vi "Dashboard Main.vi"() -> ()   [LabVIEW 2013]
uses:
  Downloads/Control 1.ctl
  <vilib>/event_ctls.llb/eventvkey.ctl
  <vilib>/Utility/file.llb/Read From Spreadsheet File (DBL).vi
panel:
  in  "Tab Control":T1(tab)
  out "Loaded":T2
  out "Armed":T2
  out "Gathering":T2
  out "Gyro":T2
  out "Flip Axes":T2
  out "Winch Power":T2
  out "Offset":dbl format="Offset: %#_g"
  out "Shot count":dbl format="%#_g shots"
  out "Offset Recieved":dbl
  in  "Jew Bar":bool=TRUE
  in  "Arm":bool=TRUE
  in  "Winch":bool=TRUE
  in  "Trigger":bool=TRUE
  in  "Intake":bool=TRUE
  in  "Rollers":bool=TRUE
  in  "Right Drive":bool=TRUE
  in  "Left Drive":bool=TRUE
  in  "Close KnightVision":bool
  in  "Open KnightVision":bool
  out "Mode":string
  out "Vision":string
  out "data out":string
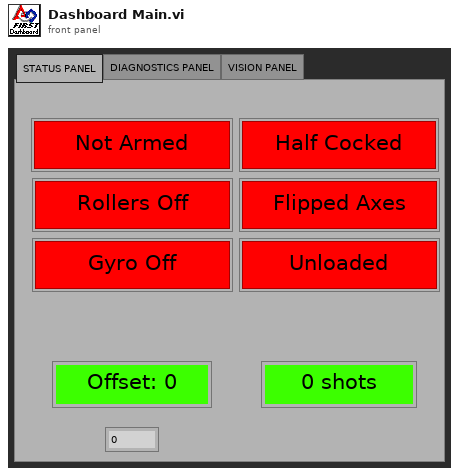
[diagram p1: front panel]
types:
  T1 = enum32{"STATUS PANEL", "DIAGNOSTICS PANEL", "VISION PANEL"}
  T2 = typedef "Control 1.ctl" = bool
  T3 = typedef "eventvkey.ctl" = enum16{"ASCII", "Enter", "Return", "Shift", "Ctrl", "Alt", "Cmd", "Opt", "Caps", "NumLock", "Clear", "Break", "Up", "Down", "Left", "Right", "Insert", "Delete", "Home", "End", "PageUp", "PageDown", "Escape", "Help", "Pause", "ScrollLock", "F1", "F2", "F3", "F4", "F5", "F6", "F7", "F8", "F9", "F10", "F11", "F12", "F13", "F14", "F15", "F16", "F17", "F18", "F19", "F20", "F21", "F22", "F23", "F24", "Play", "VolumeUp", "VolumeDown", "Mute", "Two Byte Char"}
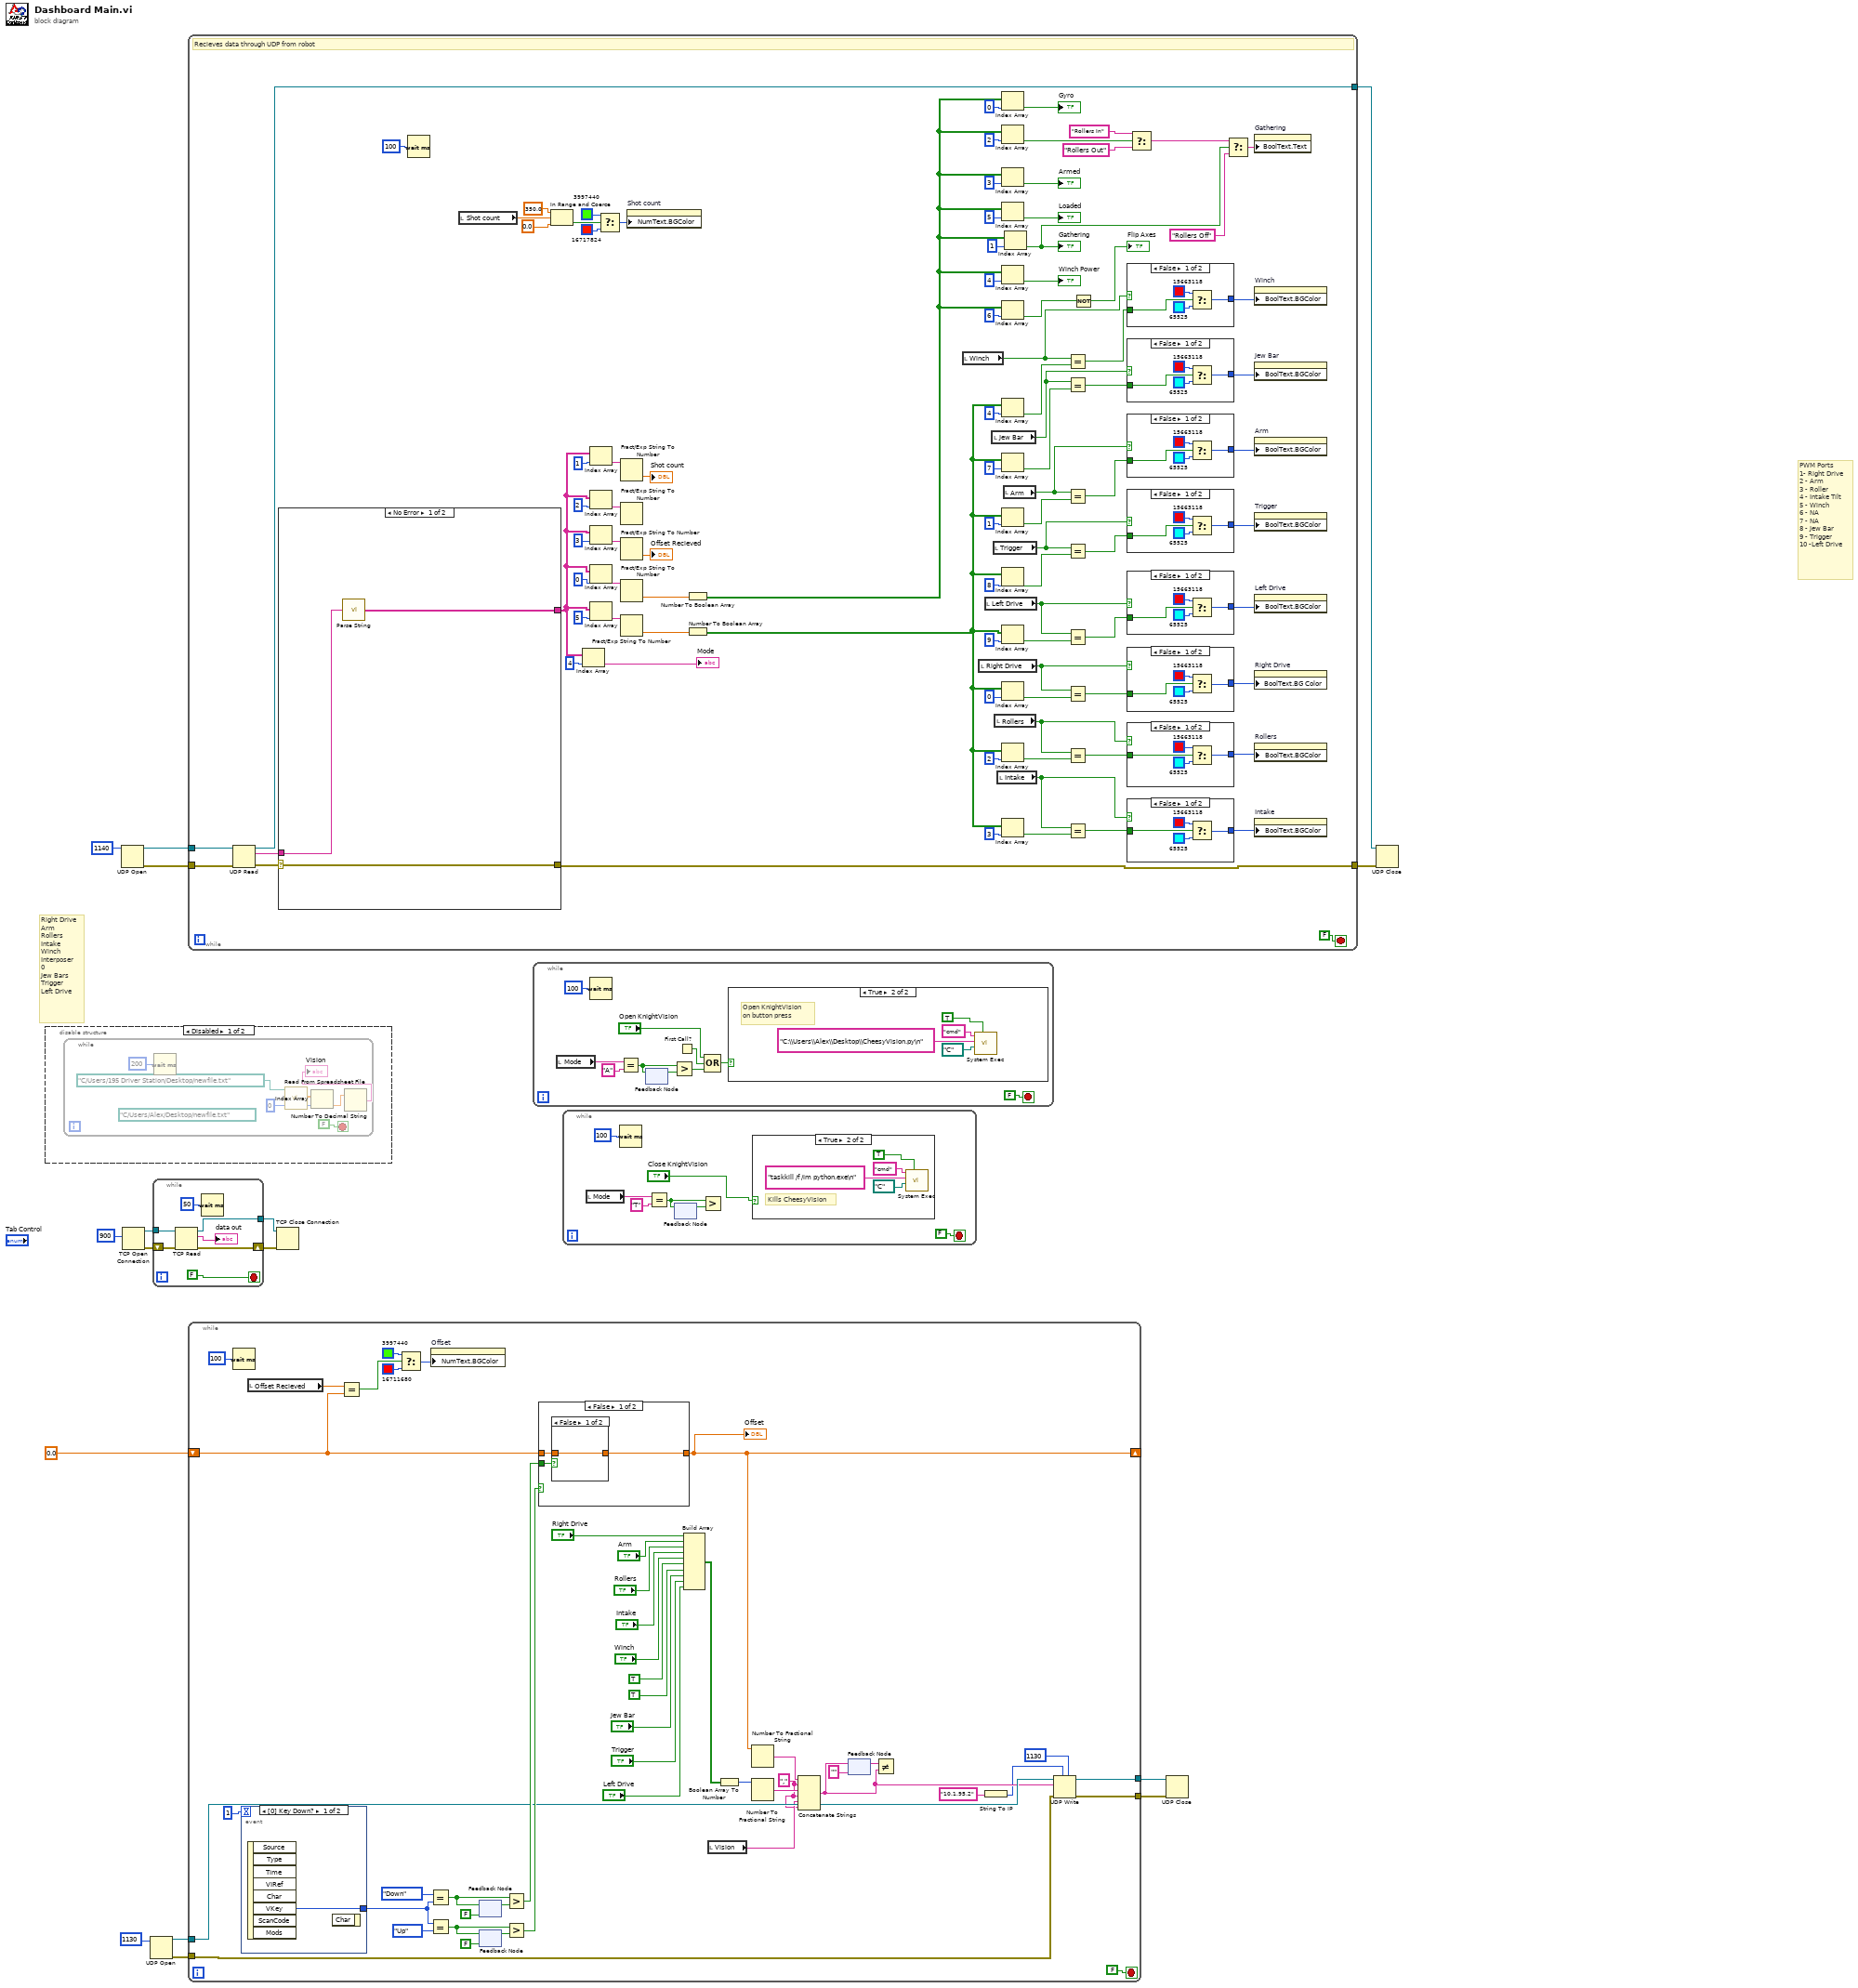
[diagram p0: block diagram]
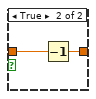
[diagram p5: hidden frame]
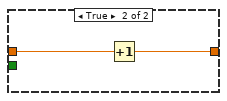
[diagram p6: hidden frame]
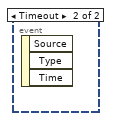
[diagram p7: hidden frame]
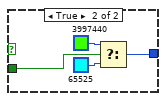
[diagram p8: hidden frame]
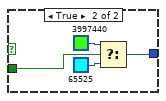
[diagram p9: hidden frame]
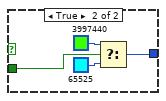
[diagram p10: hidden frame]
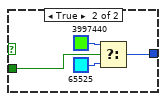
[diagram p11: hidden frame]
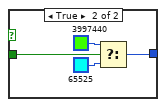
[diagram p12: hidden frame]
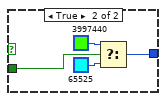
[diagram p13: hidden frame]
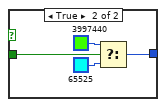
[diagram p14: hidden frame]
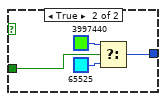
[diagram p15: hidden frame]
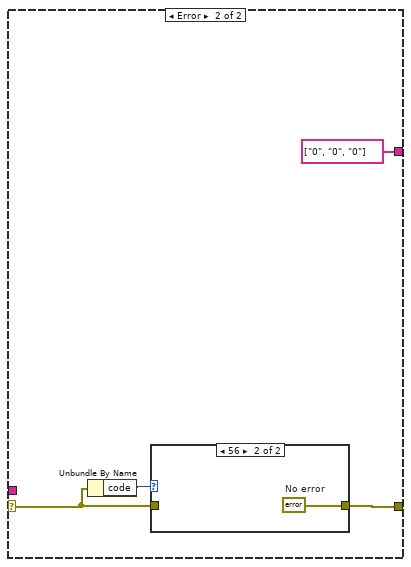
[diagram p16: hidden frame]
diagram:
  # "PWM Ports\n1- Right Drive\n2 - Arm\n3 - Roller\n4 - Intake Tilt \n5 - Winch\n6 - NA \n7 - NA\n8 - Jew Bar\n9 - Trigger\n10 -Left Drive"
  # "Right Drive\nArm\nRollers\nIntake\nWinch\nInterposer\n0\nJew Bars\nTrigger\nLeft Drive"
  n1 = disable-structure shown="Disabled" {
    frame Disabled {
      n2 = while {
        stop <- FALSE stop-if-true
        (unwired) path "C:/Users/Alex/Desktop/newfile.txt" ("file (use dialog)")
        n3 = Wait (ms)(milliseconds to wait=u32 200) -> ()  [unwired: 1 out]
        n4 = call-poly <vilib>:"Read From Spreadsheet File.vi"("file path (dialog if empty)"=path "C:/Users/195 Driver Station/Desktop/newfile.txt" ("file (use dialog)")) -> ("first row"=w21:dbl[])  [unwired: 6 in, 4 out]
        n5 = Index Array(array=w21, index=0) -> (element=w19:dbl)
        n6 = Number To Decimal String(number=w19) -> (decimal integer string=→"Vision":string)  [unwired: 1 in]
      }
    }
    frame Enabled {
    }
  }
  n7 = UDP Open(11:u16 1140) -> (port=w13:refnum<k16>, 0:w14:errorcluster)  [unwired: 4 in, 1 out]
  n8 = TCP Open Connection(remote port or service name=u16 900) -> (connection ID=w3:refnum<k5>, error out=w2:errorcluster)  [unwired: 4 in]
  n9 = UDP Open(11:u16 1130 ("port")) -> (port=w9:refnum<k16>, 0:w8:errorcluster)  [unwired: 4 in, 1 out]
  n10 = while {
    tunnel: [w29] -> w5
    tunnel: w3 -> [w27]
    shift-right: [w28] -> w4
    shift-left: w2 -> [w26]
    stop <- FALSE stop-if-true
    n11 = TCP Read(connection ID=w27, error in (no error)=w26) -> (connection ID out=w29:refnum<k5>, data out=→"data out":string, error out=w28:errorcluster)  [unwired: 3 in]
    n12 = Wait (ms)(milliseconds to wait=u32 50) -> ()  [unwired: 1 out]
  }
  n13 = while {
    tunnel: [w124] -> w16
    tunnel: [w123] -> w15
    tunnel: w14 -> [w122]
    tunnel: w13 -> [w121]
    stop <- FALSE stop-if-true
    # "Recieves data through UDP from robot"
    n14 = UDP Read(connection ID=w121, 8:w122) -> (data out=w120:string, error out=w119:errorcluster, 3:w124:refnum<k16>)  [unwired: 1 in, 3 out]
    n15 = case shown="No Error" w119 {
      selector: w119 -> [w191 w194]
      tunnel: w120 -> [w190 _]
      tunnel: [w191 w193] -> w123
      tunnel: [w189 string[] ["0", "0", "0"] ("Array Out")] -> w33
      frame No Error {
        n16 = call "Parse String.vi"("String In"=w190) -> ("Array Out"=w189:string[])
      }
      frame Error {
        n17 = Unbundle By Name(w194) -> ("code"=w195:i32)
        n18 = case shown="56" w195 {
          tunnel: w194 -> [w196 _]
          tunnel: [w196 w197] -> w193
          frame Default {
          }
          frame 56 {
            w197 = errorcluster {"status"=FALSE, "code"=0, "source"=""}  # No error
          }
        }
      }
    }
    n19 = Wait (ms)(milliseconds to wait=u32 100) -> ()  [unwired: 1 out]
    n20 = local read "Shot count"() -> (w94:dbl)
    n21 = In Range and Coerce(upper limit=350.0, x=w94, lower limit=0.0) -> (In Range?=w91:bool)  [unwired: 1 out]
    n22 = Index Array(array=w33, index=4) -> (element=→"Mode":string)
    n23 = Index Array(array=w33, index=1) -> (element=w98:string)
    n24 = Index Array(array=w33, index=2) -> (element=w99:string)
    n25 = Index Array(array=w33, index=3) -> (element=w80:string)
    n26 = Index Array(array=w33, index=0) -> (element=w116:string)
    n27 = Index Array(array=w33, index=5) -> (element=w75:string)
    n28 = Select(t=u32 3997440, s=w91, f=u32 16717824) -> (s? t:f=w78:u32)
    n29 = Fract/Exp String To Number(string=w98) -> (number=→"Shot count":dbl)  [unwired: 3 in, 1 out]
    n30 = Fract/Exp String To Number(string=w99) -> ()  [unwired: 3 in, 2 out]
    n31 = Fract/Exp String To Number(string=w80) -> (number=→"Offset Recieved":dbl)  [unwired: 3 in, 1 out]
    n32 = Fract/Exp String To Number(string=w116) -> (number=w115:dbl)  [unwired: 3 in, 1 out]
    n33 = Fract/Exp String To Number(string=w75) -> (number=w76:dbl)  [unwired: 3 in, 1 out]
    n34 = property on="Shot count" class="DigNum (strict)"("NumText.BGColor"=w78) -> ()  [unwired: 2 in, 2 out]
    n35 = Number To Boolean Array(number=w115) -> (Boolean array=w102:bool[])
    n36 = Number To Boolean Array(number=w76) -> (Boolean array=w37:bool[])
    n37 = local read "Winch"() -> (w32:bool)
    n38 = local read "Right Drive"() -> (w65:bool)
    n39 = local read "Left Drive"() -> (w42:bool)
    n40 = local read "Jew Bar"() -> (w48:bool)
    n41 = local read "Trigger"() -> (w45:bool)
    n42 = local read "Rollers"() -> (w64:bool)
    n43 = local read "Intake"() -> (w60:bool)
    n44 = Index Array(array=w102, index=0) -> (element=→"Gyro":bool)
    n45 = Index Array(array=w102, index=2) -> (element=w83:bool)
    n46 = Index Array(array=w102, index=3) -> (element=→"Armed":bool)
    n47 = Index Array(array=w102, index=5) -> (element=→"Loaded":bool)
    n48 = Index Array(array=w102, index=4) -> (element=→"Winch Power":bool)
    n49 = Index Array(array=w102, index=6) -> (element=w101:bool)
    n50 = Index Array(array=w37, index=4) -> (element=w51:bool)
    n51 = Index Array(array=w37, index=7) -> (element=w47:bool)
    n52 = Index Array(array=w37, index=1) -> (element=w58:bool)
    n53 = Index Array(array=w37, index=8) -> (element=w36:bool)
    n54 = Index Array(array=w37, index=9) -> (element=w35:bool)
    n55 = Index Array(array=w37, index=0) -> (element=w68:bool)
    n56 = Index Array(array=w37, index=2) -> (element=w56:bool)
    n57 = Index Array(array=w37, index=3) -> (element=w52:bool)
    n58 = local read "Arm"() -> (w61:bool)
    n59 = Index Array(array=w102, index=1) -> (element=w82:bool)
    "Gathering" <- w82
    n60 = Equal?(x=w32, y=w51) -> (x = y?=w53:bool)
    n61 = Equal?(x=w48, y=w47) -> (x = y?=w49:bool)
    n62 = Equal?(x=w61, y=w58) -> (x = y?=w62:bool)
    n63 = Equal?(x=w45, y=w36) -> (x = y?=w44:bool)
    n64 = Equal?(x=w42, y=w35) -> (x = y?=w43:bool)
    n65 = Equal?(x=w65, y=w68) -> (x = y?=w67:bool)
    n66 = Equal?(x=w64, y=w56) -> (x = y?=w63:bool)
    n67 = Equal?(x=w60, y=w52) -> (x = y?=w59:bool)
    n68 = Not(x=w101) -> (.not. x?=→"Flip Axes":bool)
    n69 = case shown="False" w32 {
      tunnel: w53 -> [w151 w156]
      tunnel: [w152 w153] -> w50
      frame False {
        n70 = Select(t=u32 15663118, s=w151, f=u32 65525) -> (s? t:f=w152:u32)
      }
      frame True {
        n71 = Select(t=u32 3997440, s=w156, f=u32 65525) -> (s? t:f=w153:u32)
      }
    }
    n72 = case shown="False" w48 {
      tunnel: w49 -> [w143 w148]
      tunnel: [w144 w145] -> w46
      frame False {
        n73 = Select(t=u32 15663118, s=w143, f=u32 65525) -> (s? t:f=w144:u32)
      }
      frame True {
        n74 = Select(t=u32 3997440, s=w148, f=u32 65525) -> (s? t:f=w145:u32)
      }
    }
    n75 = case shown="False" w61 {
      tunnel: w62 -> [w167 w172]
      tunnel: [w168 w169] -> w57
      frame False {
        n76 = Select(t=u32 15663118, s=w167, f=u32 65525) -> (s? t:f=w168:u32)
      }
      frame True {
        n77 = Select(t=u32 3997440, s=w172, f=u32 65525) -> (s? t:f=w169:u32)
      }
    }
    n78 = case shown="False" w45 {
      tunnel: w44 -> [w135 w140]
      tunnel: [w136 w137] -> w41
      frame False {
        n79 = Select(t=u32 15663118, s=w135, f=u32 65525) -> (s? t:f=w136:u32)
      }
      frame True {
        n80 = Select(t=u32 3997440, s=w140, f=u32 65525) -> (s? t:f=w137:u32)
      }
    }
    n81 = case shown="False" w42 {
      tunnel: w43 -> [w127 w132]
      tunnel: [w128 w129] -> w40
      frame False {
        n82 = Select(t=u32 15663118, s=w127, f=u32 65525) -> (s? t:f=w128:u32)
      }
      frame True {
        n83 = Select(t=u32 3997440, s=w132, f=u32 65525) -> (s? t:f=w129:u32)
      }
    }
    n84 = case shown="False" w65 {
      tunnel: w67 -> [w183 w188]
      tunnel: [w184 w185] -> w66
      frame False {
        n85 = Select(t=u32 15663118, s=w183, f=u32 65525) -> (s? t:f=w184:u32)
      }
      frame True {
        n86 = Select(t=u32 3997440, s=w188, f=u32 65525) -> (s? t:f=w185:u32)
      }
    }
    n87 = case shown="False" w64 {
      tunnel: w63 -> [w175 w180]
      tunnel: [w176 w177] -> w55
      frame False {
        n88 = Select(t=u32 15663118, s=w175, f=u32 65525) -> (s? t:f=w176:u32)
      }
      frame True {
        n89 = Select(t=u32 3997440, s=w180, f=u32 65525) -> (s? t:f=w177:u32)
      }
    }
    n90 = case shown="False" w60 {
      tunnel: w59 -> [w159 w164]
      tunnel: [w160 w161] -> w54
      frame False {
        n91 = Select(t=u32 15663118, s=w159, f=u32 65525) -> (s? t:f=w160:u32)
      }
      frame True {
        n92 = Select(t=u32 3997440, s=w164, f=u32 65525) -> (s? t:f=w161:u32)
      }
    }
    n93 = Select(t="Rollers In" ("Boolean Text.Text"), s=w83, f="Rollers Out" ("Boolean Text.Text")) -> (s? t:f=w84:string)
    n94 = Select(t=w84, s=w82, f="Rollers Off") -> (s? t:f=w88:string)
    n95 = property on="Gathering" class="Bool (strict)"("BoolText.Text"=w88) -> ()  [unwired: 2 in, 2 out]
    n96 = property on="Winch" class="Bool (strict)"("BoolText.BGColor"=w50) -> ()  [unwired: 2 in, 2 out]
    n97 = property on="Jew Bar" class="Bool (strict)"("BoolText.BGColor"=w46) -> ()  [unwired: 2 in, 2 out]
    n98 = property on="Arm" class="Bool (strict)"("BoolText.BGColor"=w57) -> ()  [unwired: 2 in, 2 out]
    n99 = property on="Trigger" class="Bool (strict)"("BoolText.BGColor"=w41) -> ()  [unwired: 2 in, 2 out]
    n100 = property on="Left Drive" class="Bool (strict)"("BoolText.BGColor"=w40) -> ()  [unwired: 2 in, 2 out]
    n101 = property on="Right Drive" class="Bool (strict)"("BoolText.BG Color"=w66) -> ()  [unwired: 2 in, 2 out]
    n102 = property on="Rollers" class="Bool (strict)"("BoolText.BGColor"=w55) -> ()  [unwired: 2 in, 2 out]
    n103 = property on="Intake" class="Bool (strict)"("BoolText.BGColor"=w54) -> ()  [unwired: 2 in, 2 out]
  }
  n104 = while {
    shift-right: [w222] -> _
    shift-left: 0.0 ("Offset") -> [w224]
    tunnel: w9 -> [w227]
    tunnel: w8 -> [w228]
    tunnel: [w230] -> w7
    tunnel: [w229] -> w6
    stop <- FALSE stop-if-true
    w198 = "," ("string")
    n105 = Wait (ms)(milliseconds to wait=u32 100) -> ()  [unwired: 1 out]
    n106 = event shown="[0] Key Down?" {
      selector: _ -> [_ _]
      dyn-events: _ -> [_ _]
      timeout: 1 -> [_ _]
      tunnel: [w253 _] -> w236
      event Key Down? {
        n107 = event-data() -> ("VKey"=w253:T3)  [unwired: 1 in, 7 out]
        n108 = event-data() -> ()  [unwired: 2 in, 1 out]
      }
      event Timeout {
        n109 = event-data() -> ()  [unwired: 1 in, 3 out]
      }
    }
    n110 = local read "Offset Recieved"() -> (w223:dbl)
    n111 = Equal?(x=w223, y=w224) -> (x = y?=w219:bool)
    n112 = Select(t=u32 3997440, s=w219, f=u32 16711680) -> (s? t:f=w220:u32)
    n113 = Equal?(x=eventvkey."Down" ("y"), y=w236) -> (x = y?=w233:bool)
    n114 = Equal?(x=w236, y=eventvkey."Up") -> (x = y?=w239:bool)
    n115 = property on="Offset" class="DigNum (strict)"("NumText.BGColor"=w220) -> ()  [unwired: 2 in, 2 out]
    n116 = feedback #1(FALSE) -> (w234:bool)
    n117 = feedback-in #1(w233) -> ()
    n118 = feedback-in #2(w239) -> ()
    n119 = feedback #2(FALSE) -> (w240:bool)
    n120 = Greater?(x=w233, y=w234) -> (0:w231:bool)
    n121 = Greater?(x=w239, y=w240) -> (0:w237:bool)
    n122 = case shown="False" w237 {
      tunnel: [w245 w251] -> w222
      tunnel: w224 -> [w246 w252]
      tunnel: w231 -> [w247 _]
      frame False {
        n123 = case shown="False" w247 {
          tunnel: w246 -> [w248 w249]
          tunnel: [w248 w250] -> w245
          frame False {
          }
          frame True {
            n124 = Decrement(x=w249) -> (x-1=w250:dbl)
          }
        }
      }
      frame True {
        n125 = Increment(x=w252) -> (x+1=w251:dbl)
      }
    }
    "Offset" <- w222
    n126 = Build Array("Right Drive", "Arm", "Rollers", "Intake", "Winch", TRUE ("element"), TRUE ("element"), "Jew Bar", "Trigger", "Left Drive") -> (w209:bool[])
    n127 = local read "Vision"() -> (w202:string)
    n128 = Boolean Array To Number(Boolean array=w209) -> (number=w207:u32)
    n129 = Number To Fractional String(number=w222) -> (F-format string=w208:string)  [unwired: 3 in]
    n130 = Number To Fractional String(number=w207) -> (F-format string=w206:string)  [unwired: 3 in]
    n131 = Concatenate Strings(w208, w198, w206, w198, w202, w198) -> (w205:string)
    n132 = feedback-in #3(w205) -> ()
    n133 = feedback #3("") -> (w221:string)
    n134 = Not Equal?(x=w221, y=w205) -> ()  [unwired: 1 out]
    n135 = String To IP(1:"10.1.95.2" ("name")) -> (0:w201:u32)
    n136 = UDP Write(address=w201, port or service name=u16 1130, connection ID=w227, data in=w205, 8:w228) -> (error out=w229:errorcluster, 3:w230:refnum<k16>)  [unwired: 1 in]
  }
  n137 = TCP Close Connection(connection ID=w5, error in (no error)=w4) -> ()  [unwired: 1 in, 2 out]
  n138 = while {
    stop <- FALSE stop-if-true
    n139 = local read "Mode"() -> (w258:string)
    n140 = Wait (ms)(milliseconds to wait=u32 100) -> ()  [unwired: 1 out]
    n141 = Equal?(x=w258, y="A") -> (x = y?=w260:bool)
    n142 = feedback #4() -> (w261:bool)  [unwired: 1 in]
    n143 = feedback-in #4(w260) -> ()
    n144 = Greater?(x=w260, y=w261) -> (0:w255:bool)
    n145 = First Call?() -> (First Call?: T/F=w256:bool)
    n146 = Compound Arithmetic op=OR("Open KnightVision", w256, w255) -> (w254:bool)
    n147 = case shown="True" w254 {
      frame False {
      }
      frame True {
        # "Open KnightVision\non button press"
        n148 = call <vilib>:"System Exec.vi"("wait until completion? (T)"=TRUE, "working directory"=path "C:/", "standard input"="C:\\Users\\Alex\\Desktop\\CheesyVision.py\n" ("command line"), "command line"="cmd") -> ()  [unwired: 4 in, 4 out]
      }
    }
  }
  n149 = while {
    stop <- FALSE stop-if-true
    n150 = local read "Mode"() -> (w272:string)
    n151 = Wait (ms)(milliseconds to wait=u32 100) -> ()  [unwired: 1 out]
    n152 = Equal?(x=w272, y="T") -> (x = y?=w270:bool)
    n153 = feedback #5() -> (w269:bool)  [unwired: 1 in]
    n154 = feedback-in #5(w270) -> ()
    n155 = Greater?(x=w270, y=w269) -> ()  [unwired: 1 out]
    n156 = case shown="True" "Close KnightVision" {
      frame False {
      }
      frame True {
        # "Kills CheesyVision"
        n157 = call <vilib>:"System Exec.vi"("wait until completion? (T)"=TRUE, "working directory"=path "C:/", "standard input"="taskkill /f /im python.exe\n", "command line"="cmd") -> ()  [unwired: 4 in, 4 out]
      }
    }
  }
  n158 = UDP Close(connection ID=w7, 8:w6) -> ()  [unwired: 2 out]
  n159 = UDP Close(connection ID=w16, 8:w15) -> ()  [unwired: 2 out]
